vi "Abadines_server_sight.vi"() -> ()   [LabVIEW 2013]
uses:
  <vilib>/NXT/Block Support/NXT_InputPort.ctl
  <vilib>/NXT/Block Support/NXT_MessageMailbox.ctl
  <vilib>/NXT/Block Support/NXT_OutputPort.ctl
  <vilib>/NXT/Subs/MotorOutput.ctl
  <vilib>/NXT/Dual Mode Library/BT/BlueTooth_Write_Num.vi
  <vilib>/NXT/NXTIO Xnodes/NXTIONodeSubVIs/NXTStopMotors.vi
  <vilib>/NXT/Dual Mode Library/Display/drawNumber.vi
  <vilib>/NXT/Dual Mode Library/Display/drawNumber_float.vi
  <vilib>/NXT/NXTIO Xnodes/AddressXNode/NXTIOAddress.xnode
  <vilib>/NXT/NXTIO Xnodes/NXTIOXNode/NXTIO.xnode
  <vilib>/NXT/Subs/LVHSConnector.ctl
  <vilib>/NXT/LegoClasses/BrickReference/BrickReference.lvclass
panel:
  in  "threshold steer":dbl
  out "norm dist":dbl
  out "Blue Line":i16
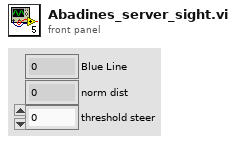
[diagram p1: front panel]
types:
  T1 = typedef "NXT_OutputPort.ctl" = u8
  T2 = typedef "NXT_InputPort.ctl" = u32
  T3 = typedef "LVHSConnector.ctl" = refnum<class "BrickReference.lvclass">
  T4 = typedef "NXT_MessageMailbox.ctl" = u8
  T5 = typedef "MotorOutput.ctl" = u8
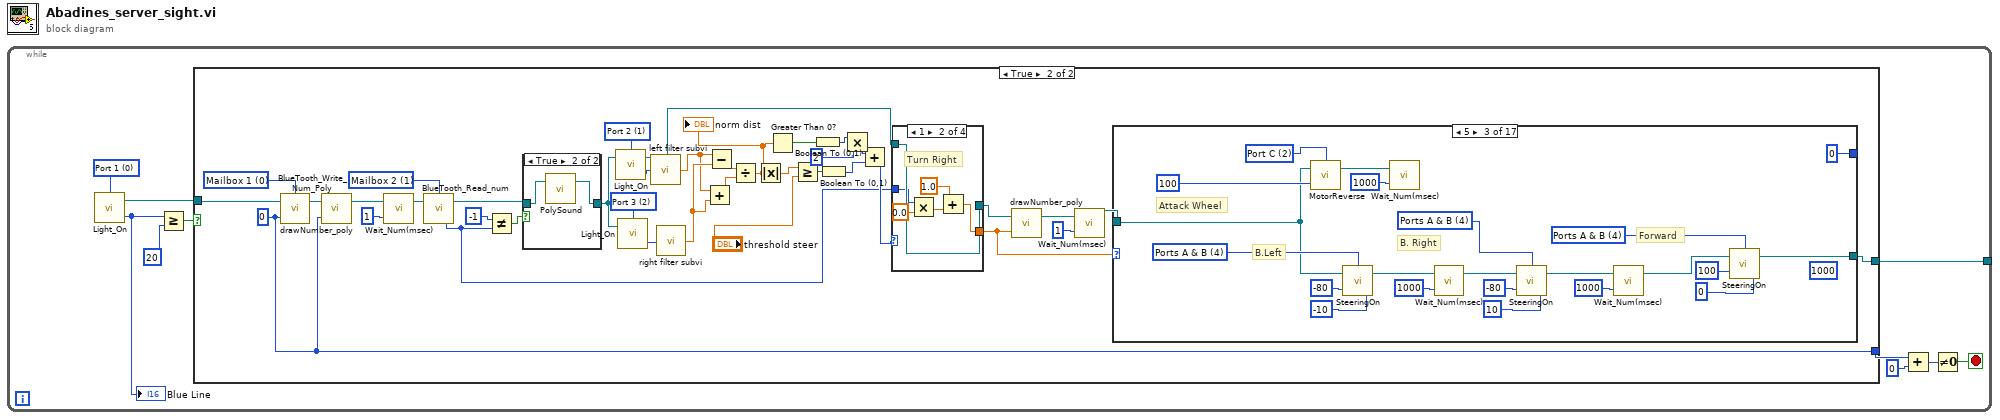
[diagram p0: block diagram]
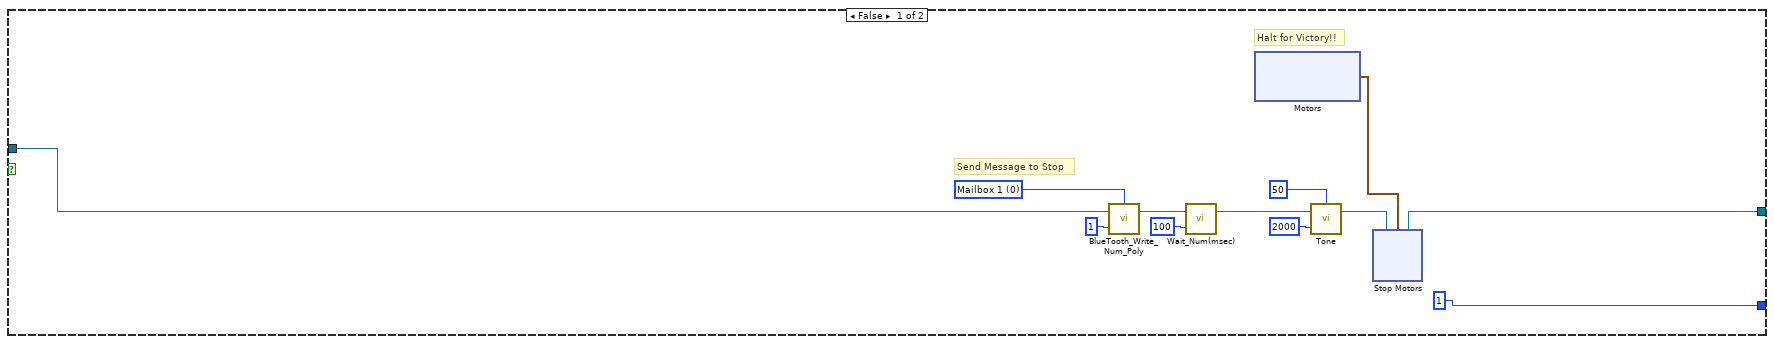
[diagram p2: hidden frame]
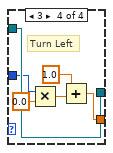
[diagram p5: hidden frame]
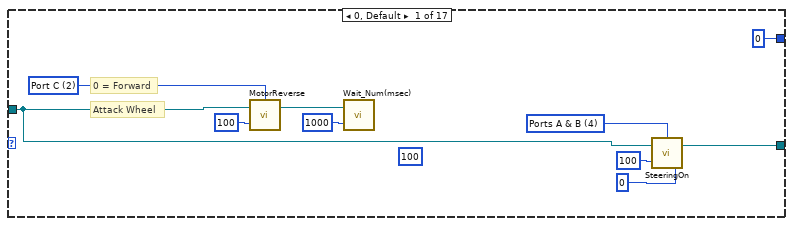
[diagram p7: hidden frame]
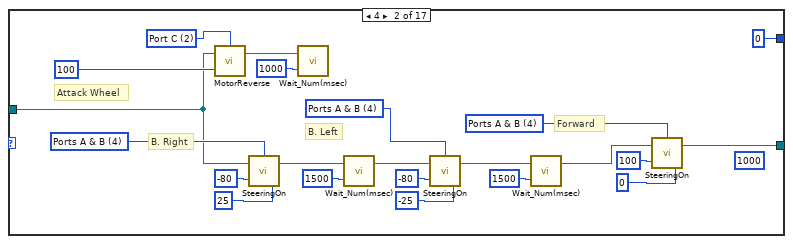
[diagram p8: hidden frame]
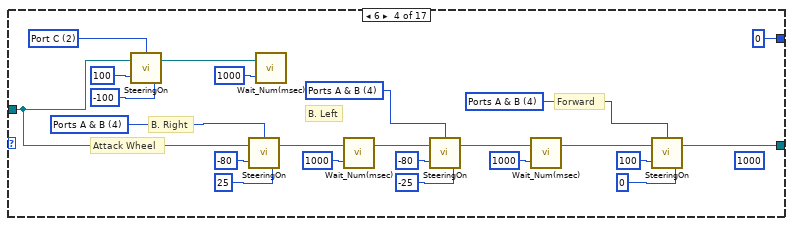
[diagram p9: hidden frame]
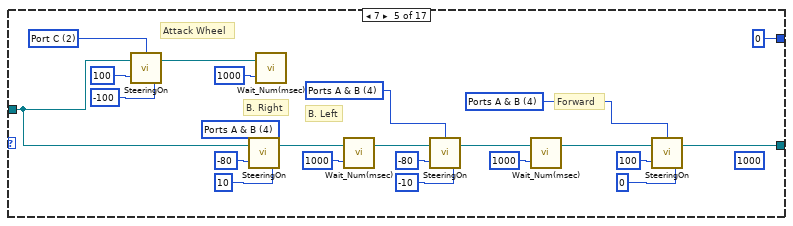
[diagram p10: hidden frame]
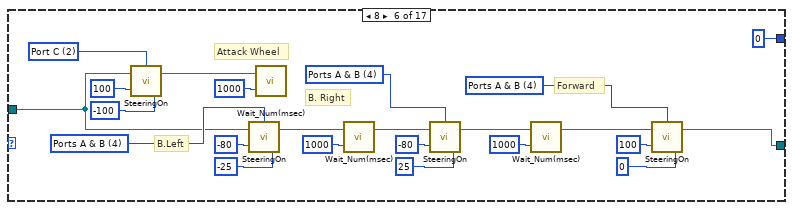
[diagram p11: hidden frame]
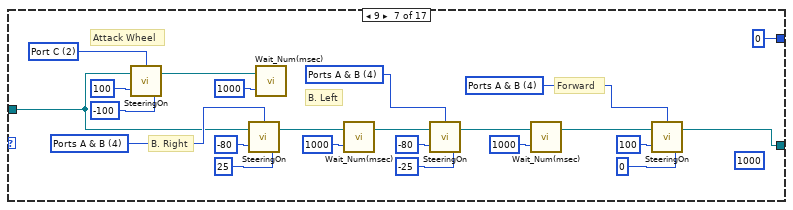
[diagram p12: hidden frame]
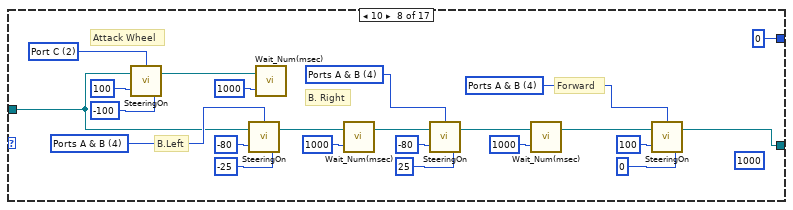
[diagram p13: hidden frame]
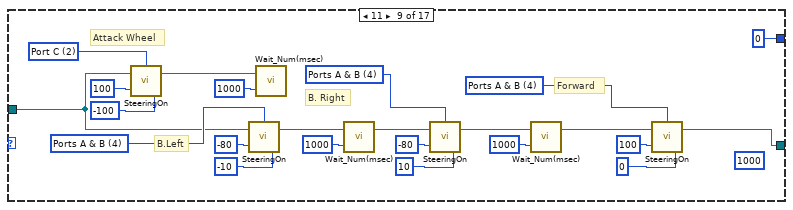
[diagram p14: hidden frame]
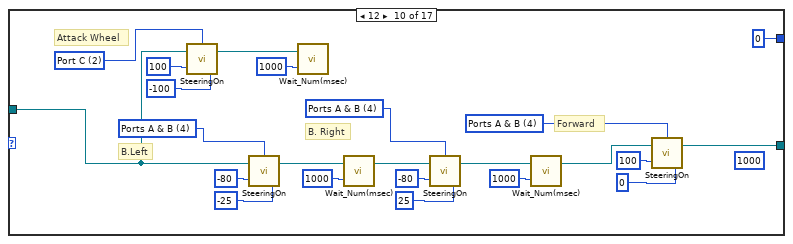
[diagram p15: hidden frame]
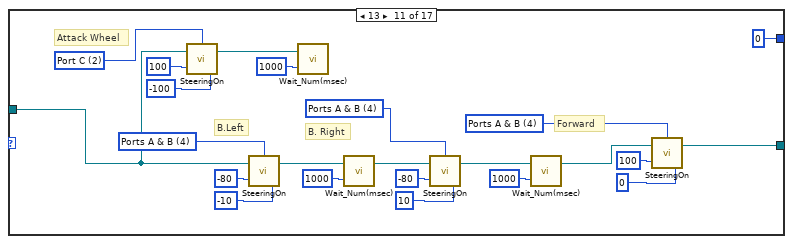
[diagram p16: hidden frame]
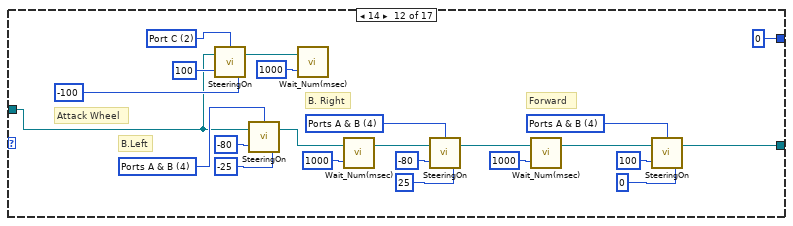
[diagram p17: hidden frame]
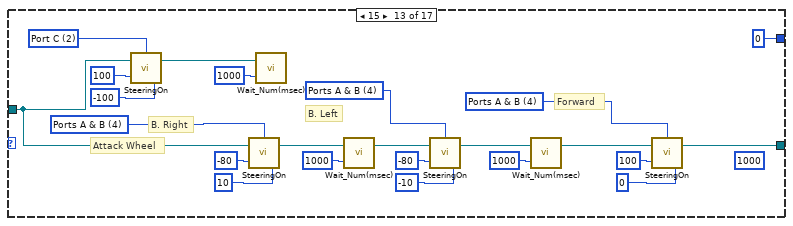
[diagram p18: hidden frame]
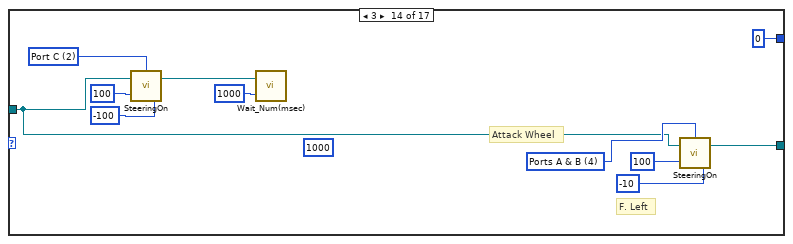
[diagram p19: hidden frame]
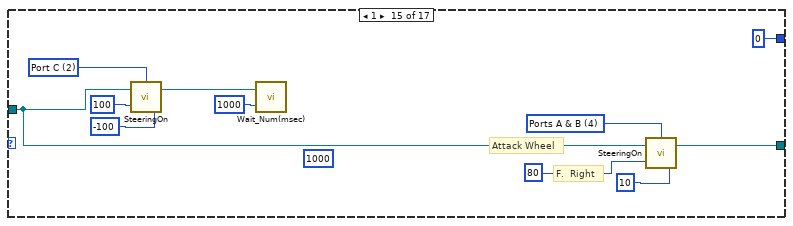
[diagram p20: hidden frame]
diagram:
  n1 = while {
    tunnel: [w6] -> _
    stop <- w2 stop-if-true
    w10 = T2 0 items=["Port 1", "Port 2", "Port 3", "Port 4"] ("Port (Port 3)")
    n2 = call <vilib>:"Light_On.vi"("Port (Port 3)"=w10) -> ("Scaled Value"=w9:i16, "NXT/EV3"=w1:T3)  [unwired: 2 in]
    "Blue Line" <- w9
    n3 = Greater Or Equal?(x=w9, y=i16 20) -> (x >= y?=w7:bool)
    n4 = case shown="True" w7 {
      tunnel: w1 -> [w20 w59]
      tunnel: [w14 w57] -> w6
      tunnel: [1 w56] -> w5
      frame False {
        w21 = T4 0 items=["Mailbox 1", "Mailbox 2", "Mailbox 3", "Mailbox 4", "Mailbox 5", "Mailbox 6", "Mailbox 7", "Mailbox 8", "Mailbox 9", "Mailbox 10"] ("Mailbox")
        # "Halt for Victory!!"
        # "Send Message to Stop"
        n5 = call-poly <vilib>:"BlueTooth_Write_Num_Poly.vi"("Message"=1, "NXT/EV3"=w20, "Mailbox"=w21) -> ("NXT/EV3"=w16:T3)  [unwired: 1 in]
        n6 = call <vilib>:"Wait_Num(msec).vi"("Time (100 msec)"=u32 100, "NXT/EV3"=w16) -> ("NXT/EV3"=w17:T3)  [unwired: 2 in]
        n7 = xnode "Motors"() -> ("Motor"=w13:cluster{"Port":T1, "Port":T1})
        n8 = call <vilib>:"Tone.vi"("Duration (500 ms)"=u16 2000, "NXT/EV3"=w17, "Tone (440 Hz)"=u16 50) -> ("NXT/EV3"=w15:T3)  [unwired: 1 in]
        n9 = xnode "Stop Motors"("Motors"=w13, "NXT/EV3"=w15) -> ("NXT/EV3"=w14:T3)
      }
      frame True {
        w50 = T2 2 items=["Port 1", "Port 2", "Port 3", "Port 4"] ("Port (Port 3)")
        w51 = T2 1 items=["Port 1", "Port 2", "Port 3", "Port 4"] ("Port (Port 3)")
        w66 = T4 1 items=["Mailbox 1", "Mailbox 2", "Mailbox 3", "Mailbox 4", "Mailbox 5", "Mailbox 6", "Mailbox 7", "Mailbox 8", "Mailbox 9", "Mailbox 10"] ("Mailbox")
        w56 = 0 ("Message")
        w60 = T4 0 items=["Mailbox 1", "Mailbox 2", "Mailbox 3", "Mailbox 4", "Mailbox 5", "Mailbox 6", "Mailbox 7", "Mailbox 8", "Mailbox 9", "Mailbox 10"] ("Mailbox")
        n10 = call-poly <vilib>:"BlueTooth_Write_Num_Poly.vi"("Message"=w56, "NXT/EV3"=w59, "Mailbox"=w60) -> ("NXT/EV3"=w53:T3)  [unwired: 1 in]
        n11 = call-poly <vilib>:"drawNumber_poly.vi"("number"=w56, "NXT/EV3"=w53) -> ("NXT/EV3"=w61:T3)  [unwired: 2 in]
        n12 = call <vilib>:"Wait_Num(msec).vi"("Time (100 msec)"=u32 1, "NXT/EV3"=w61) -> ("NXT/EV3"=w62:T3)  [unwired: 2 in]
        n13 = call <vilib>:"BlueTooth_Read_num.vi"("NXT/EV3"=w62, "Mailbox"=w66) -> ("Message"=w30:i32, "NXT/EV3"=w52:T3)  [unwired: 1 in]
        n14 = Not Equal?(x=-1, y=w30) -> (x != y?=w54:bool)
        n15 = case shown="True" w54 {
          tunnel: [w83 w85] -> w33
          tunnel: w52 -> [w83 w84]
          frame False {
          }
          frame True {
            n16 = call-poly <vilib>:"PolySound.vi"("NXT/EV3"=w84) -> ("NXT/EV3"=w85:T3)  [unwired: 3 in]
          }
        }
        n17 = call <vilib>:"Light_On.vi"("NXT/EV3"=w33, "Port (Port 3)"=w51) -> ("Scaled Value"=w48:i16, "NXT/EV3"=w32:T3)  [unwired: 1 in]
        n18 = call <vilib>:"Light_On.vi"("NXT/EV3"=w33, "Port (Port 3)"=w50) -> ("Scaled Value"=w49:i16)  [unwired: 1 in, 1 out]
        n19 = call "left filter subvi.vi"("raw value in"=w48) -> ("filtered signal"=w46:dbl)  [unwired: 14 in]
        n20 = call "right filter subvi.vi"("raw value in"=w49) -> ("filtered signal"=w47:dbl)  [unwired: 14 in]
        n21 = Add(x=w46, y=w47) -> (x+y=w44:dbl)
        n22 = Subtract(x=w46, y=w47) -> (x-y=w45:dbl)
        n23 = Divide(x=w45, y=w44) -> (x/y=w41:dbl)
        "norm dist" <- w41
        n24 = Absolute Value(x=w41) -> (abs(x)=w43:dbl)
        n25 = Greater Than 0?(x=w41) -> (x > 0?=w39:bool)
        n26 = Greater Or Equal?(x=w43, y="threshold steer") -> (x >= y?=w40:bool)
        n27 = Boolean To (0,1)(Boolean=w39) -> (0, 1=w38:i16)
        n28 = Boolean To (0,1)(Boolean=w40) -> (0, 1=w36:i16)
        n29 = Multiply(x=w38, y=i16 2) -> (x*y=w35:i16)
        n30 = Add(x=w35, y=w36) -> (x+y=w34:i16)
        n31 = case shown="1" w34 {
          tunnel: w32 -> [w68 w72 w76 w82]
          tunnel: [w68 w72 w76 w82] -> w31
          tunnel: w30 -> [w67 w71 w75 w78]
          tunnel: [w67 w70 w75 w77] -> w29
          frame 0, Default {
          }
          frame 1 {
            # "Turn Right"
            n32 = Multiply(x=w71, y=0.0) -> (x*y=w69:dbl)
            n33 = Add(x=1.0, y=w69) -> (x+y=w70:dbl)
          }
          frame 2 {
          }
          frame 3 {
            # "Turn Left"
            n34 = Multiply(x=w78, y=0.0) -> (x*y=w80:dbl)
            n35 = Add(x=1.0, y=w80) -> (x+y=w77:dbl)
          }
        }
        n36 = call-poly <vilib>:"drawNumber_poly.vi"("number"=w29, "NXT/EV3"=w31) -> ("NXT/EV3"=w65:T3)  [unwired: 2 in]
        n37 = call <vilib>:"Wait_Num(msec).vi"("Time (100 msec)"=u32 1, "NXT/EV3"=w65) -> ("NXT/EV3"=w58:T3)  [unwired: 2 in]
        n38 = case shown="5" w29 {
          tunnel: [w93 w111 w124 w147 w170 w202 w216 w239 w262 w286 w308 w331 w355 w378 w389 w398 w415] -> w57
          tunnel: w58 -> [w86 w96 w118 w140 w163 w186 w209 w232 w255 w279 w302 w324 w347 w370 w381 w394 w408]
          tunnel: [0 ("Steering (100)") 0 ("Steering (100)") 0 ("Steering (100)") 0 ("Steering (100)") 0 ("Steering (100)") 0 ("Steering (100)") 0 ("Steering (100)") 0 ("Steering (100)") 0 ("Steering (100)") 0 ("Steering (100)") 0 ("Steering (100)") 0 ("Steering (100)") 0 ("Steering (100)") 0 ("Steering (100)") 0 ("Steering (100)") 1 ("Steering (100)") 0 ("Steering (100)")] -> _
          frame 0, Default {
            (unwired) u16 100 ("Duration (500 ms)")
            w91 = T5 2 items=["Port A"=0, "Port B"=1, "Port C"=2, "Ports A & B"=4, "Ports A & C"=5, "Ports B & C"=6, "All Ports"=3] ("Output Ports (A & B)")
            w92 = T5 4 items=["Port A"=0, "Port B"=1, "Port C"=2, "Ports A & B"=4, "Ports A & C"=5, "Ports B & C"=6, "All Ports"=3] ("Output Ports (A & B) 5")
            # "Attack Wheel"
            # "0 = Forward"
            n39 = call <vilib>:"MotorReverse.vi"("Power (75)"=100, "NXT/EV3"=w86, "Output Port (All Ports)"=w91) -> ("NXT/EV3"=w89:T3)  [unwired: 1 in]
            n40 = call <vilib>:"Wait_Num(msec).vi"("Time (100 msec)"=u32 1000, "NXT/EV3"=w89) -> ()  [unwired: 2 in, 1 out]
            n41 = call <vilib>:"SteeringOn.vi"("Power (75)"=100, "Steering (100)"=0, "NXT/EV3"=w86, "Output Ports (A & B)"=w92) -> ("NXT/EV3"=w93:T3)
          }
          frame 4 {
            (unwired) u16 1000 ("Duration (500 ms)")
            w101 = T5 2 items=["Port A"=0, "Port B"=1, "Port C"=2, "Ports A & B"=4, "Ports A & C"=5, "Ports B & C"=6, "All Ports"=3] ("Output Ports (A & B)")
            w108 = T5 4 items=["Port A"=0, "Port B"=1, "Port C"=2, "Ports A & B"=4, "Ports A & C"=5, "Ports B & C"=6, "All Ports"=3] ("Output Ports (A & B) 15")
            w109 = T5 4 items=["Port A"=0, "Port B"=1, "Port C"=2, "Ports A & B"=4, "Ports A & C"=5, "Ports B & C"=6, "All Ports"=3] ("Output Port (All Ports) 6")
            w110 = T5 4 items=["Port A"=0, "Port B"=1, "Port C"=2, "Ports A & B"=4, "Ports A & C"=5, "Ports B & C"=6, "All Ports"=3] ("Output Ports (A & B) 16")
            # "Attack Wheel"
            # "Forward"
            # "B. Left"
            # "B. Right"
            n42 = call <vilib>:"MotorReverse.vi"("Power (75)"=100, "NXT/EV3"=w96, "Output Port (All Ports)"=w101) -> ("NXT/EV3"=w99:T3)  [unwired: 1 in]
            n43 = call <vilib>:"SteeringOn.vi"("Power (75)"=-80, "Steering (100)"=25, "NXT/EV3"=w96, "Output Ports (A & B)"=w110) -> ("NXT/EV3"=w107:T3)
            n44 = call <vilib>:"Wait_Num(msec).vi"("Time (100 msec)"=u32 1000, "NXT/EV3"=w99) -> ()  [unwired: 2 in, 1 out]
            n45 = call <vilib>:"Wait_Num(msec).vi"("Time (100 msec)"=u32 1500, "NXT/EV3"=w107) -> ("NXT/EV3"=w106:T3)  [unwired: 2 in]
            n46 = call <vilib>:"SteeringOn.vi"("Power (75)"=-80, "Steering (100)"=-25, "NXT/EV3"=w106, "Output Ports (A & B)"=w109) -> ("NXT/EV3"=w105:T3)
            n47 = call <vilib>:"Wait_Num(msec).vi"("Time (100 msec)"=u32 1500, "NXT/EV3"=w105) -> ("NXT/EV3"=w104:T3)  [unwired: 2 in]
            n48 = call <vilib>:"SteeringOn.vi"("Power (75)"=100, "Steering (100)"=0, "NXT/EV3"=w104, "Output Ports (A & B)"=w108) -> ("NXT/EV3"=w111:T3)
          }
          frame 5 {
            (unwired) u16 1000 ("Duration (500 ms)")
            w123 = T5 2 items=["Port A"=0, "Port B"=1, "Port C"=2, "Ports A & B"=4, "Ports A & C"=5, "Ports B & C"=6, "All Ports"=3] ("Output Ports (A & B)")
            w131 = T5 4 items=["Port A"=0, "Port B"=1, "Port C"=2, "Ports A & B"=4, "Ports A & C"=5, "Ports B & C"=6, "All Ports"=3] ("Output Ports (A & B) 21")
            w132 = T5 4 items=["Port A"=0, "Port B"=1, "Port C"=2, "Ports A & B"=4, "Ports A & C"=5, "Ports B & C"=6, "All Ports"=3] ("Output Port (All Ports) 9")
            w133 = T5 4 items=["Port A"=0, "Port B"=1, "Port C"=2, "Ports A & B"=4, "Ports A & C"=5, "Ports B & C"=6, "All Ports"=3] ("Output Ports (A & B) 22")
            # "Attack Wheel"
            # "Forward"
            # "B. Right"
            # "B.Left"
            n49 = call <vilib>:"MotorReverse.vi"("Power (75)"=100, "NXT/EV3"=w118, "Output Port (All Ports)"=w123) -> ("NXT/EV3"=w121:T3)  [unwired: 1 in]
            n50 = call <vilib>:"SteeringOn.vi"("Power (75)"=-80, "Steering (100)"=-10, "NXT/EV3"=w118, "Output Ports (A & B)"=w133) -> ("NXT/EV3"=w129:T3)
            n51 = call <vilib>:"Wait_Num(msec).vi"("Time (100 msec)"=u32 1000, "NXT/EV3"=w121) -> ()  [unwired: 2 in, 1 out]
            n52 = call <vilib>:"Wait_Num(msec).vi"("Time (100 msec)"=u32 1000, "NXT/EV3"=w129) -> ("NXT/EV3"=w128:T3)  [unwired: 2 in]
            n53 = call <vilib>:"SteeringOn.vi"("Power (75)"=-80, "Steering (100)"=10, "NXT/EV3"=w128, "Output Ports (A & B)"=w132) -> ("NXT/EV3"=w126:T3)
            n54 = call <vilib>:"Wait_Num(msec).vi"("Time (100 msec)"=u32 1000, "NXT/EV3"=w126) -> ("NXT/EV3"=w125:T3)  [unwired: 2 in]
            n55 = call <vilib>:"SteeringOn.vi"("Power (75)"=100, "Steering (100)"=0, "NXT/EV3"=w125, "Output Ports (A & B)"=w131) -> ("NXT/EV3"=w124:T3)
          }
          frame 6 {
            (unwired) u16 1000 ("Duration (500 ms)")
            w146 = T5 2 items=["Port A"=0, "Port B"=1, "Port C"=2, "Ports A & B"=4, "Ports A & C"=5, "Ports B & C"=6, "All Ports"=3] ("Output Ports (A & B)")
            w156 = T5 4 items=["Port A"=0, "Port B"=1, "Port C"=2, "Ports A & B"=4, "Ports A & C"=5, "Ports B & C"=6, "All Ports"=3] ("Output Ports (A & B) 15")
            w155 = T5 4 items=["Port A"=0, "Port B"=1, "Port C"=2, "Ports A & B"=4, "Ports A & C"=5, "Ports B & C"=6, "All Ports"=3] ("Output Port (All Ports) 6")
            w154 = T5 4 items=["Port A"=0, "Port B"=1, "Port C"=2, "Ports A & B"=4, "Ports A & C"=5, "Ports B & C"=6, "All Ports"=3] ("Output Ports (A & B) 16")
            # "Attack Wheel"
            # "Forward"
            # "B. Left"
            # "B. Right"
            n56 = call <vilib>:"SteeringOn.vi"("Power (75)"=100, "Steering (100)"=-100, "NXT/EV3"=w140, "Output Ports (A & B)"=w146) -> ("NXT/EV3"=w143:T3)
            n57 = call <vilib>:"SteeringOn.vi"("Power (75)"=-80, "Steering (100)"=25, "NXT/EV3"=w140, "Output Ports (A & B)"=w154) -> ("NXT/EV3"=w157:T3)
            n58 = call <vilib>:"Wait_Num(msec).vi"("Time (100 msec)"=u32 1000, "NXT/EV3"=w143) -> ()  [unwired: 2 in, 1 out]
            n59 = call <vilib>:"Wait_Num(msec).vi"("Time (100 msec)"=u32 1000, "NXT/EV3"=w157) -> ("NXT/EV3"=w158:T3)  [unwired: 2 in]
            n60 = call <vilib>:"SteeringOn.vi"("Power (75)"=-80, "Steering (100)"=-25, "NXT/EV3"=w158, "Output Ports (A & B)"=w155) -> ("NXT/EV3"=w159:T3)
            n61 = call <vilib>:"Wait_Num(msec).vi"("Time (100 msec)"=u32 1000, "NXT/EV3"=w159) -> ("NXT/EV3"=w160:T3)  [unwired: 2 in]
            n62 = call <vilib>:"SteeringOn.vi"("Power (75)"=100, "Steering (100)"=0, "NXT/EV3"=w160, "Output Ports (A & B)"=w156) -> ("NXT/EV3"=w147:T3)
          }
          frame 7 {
            (unwired) u16 1000 ("Duration (500 ms)")
            w169 = T5 2 items=["Port A"=0, "Port B"=1, "Port C"=2, "Ports A & B"=4, "Ports A & C"=5, "Ports B & C"=6, "All Ports"=3] ("Output Ports (A & B)")
            w179 = T5 4 items=["Port A"=0, "Port B"=1, "Port C"=2, "Ports A & B"=4, "Ports A & C"=5, "Ports B & C"=6, "All Ports"=3] ("Output Ports (A & B) 15")
            w178 = T5 4 items=["Port A"=0, "Port B"=1, "Port C"=2, "Ports A & B"=4, "Ports A & C"=5, "Ports B & C"=6, "All Ports"=3] ("Output Port (All Ports) 6")
            w177 = T5 4 items=["Port A"=0, "Port B"=1, "Port C"=2, "Ports A & B"=4, "Ports A & C"=5, "Ports B & C"=6, "All Ports"=3] ("Output Ports (A & B) 16")
            # "Attack Wheel"
            # "Forward"
            # "B. Left"
            # "B. Right"
            n63 = call <vilib>:"SteeringOn.vi"("Power (75)"=100, "Steering (100)"=-100, "NXT/EV3"=w163, "Output Ports (A & B)"=w169) -> ("NXT/EV3"=w166:T3)
            n64 = call <vilib>:"SteeringOn.vi"("Power (75)"=-80, "Steering (100)"=10, "NXT/EV3"=w163, "Output Ports (A & B)"=w177) -> ("NXT/EV3"=w180:T3)
            n65 = call <vilib>:"Wait_Num(msec).vi"("Time (100 msec)"=u32 1000, "NXT/EV3"=w166) -> ()  [unwired: 2 in, 1 out]
            n66 = call <vilib>:"Wait_Num(msec).vi"("Time (100 msec)"=u32 1000, "NXT/EV3"=w180) -> ("NXT/EV3"=w181:T3)  [unwired: 2 in]
            n67 = call <vilib>:"SteeringOn.vi"("Power (75)"=-80, "Steering (100)"=-10, "NXT/EV3"=w181, "Output Ports (A & B)"=w178) -> ("NXT/EV3"=w182:T3)
            n68 = call <vilib>:"Wait_Num(msec).vi"("Time (100 msec)"=u32 1000, "NXT/EV3"=w182) -> ("NXT/EV3"=w183:T3)  [unwired: 2 in]
            n69 = call <vilib>:"SteeringOn.vi"("Power (75)"=100, "Steering (100)"=0, "NXT/EV3"=w183, "Output Ports (A & B)"=w179) -> ("NXT/EV3"=w170:T3)
          }
          frame 8 {
            w192 = T5 2 items=["Port A"=0, "Port B"=1, "Port C"=2, "Ports A & B"=4, "Ports A & C"=5, "Ports B & C"=6, "All Ports"=3] ("Output Ports (A & B)")
            w199 = T5 4 items=["Port A"=0, "Port B"=1, "Port C"=2, "Ports A & B"=4, "Ports A & C"=5, "Ports B & C"=6, "All Ports"=3] ("Output Ports (A & B) 21")
            w200 = T5 4 items=["Port A"=0, "Port B"=1, "Port C"=2, "Ports A & B"=4, "Ports A & C"=5, "Ports B & C"=6, "All Ports"=3] ("Output Port (All Ports) 9")
            w201 = T5 4 items=["Port A"=0, "Port B"=1, "Port C"=2, "Ports A & B"=4, "Ports A & C"=5, "Ports B & C"=6, "All Ports"=3] ("Output Ports (A & B) 22")
            # "Attack Wheel"
            # "Forward"
            # "B. Right"
            # "B.Left"
            n70 = call <vilib>:"SteeringOn.vi"("Power (75)"=100, "Steering (100)"=-100, "NXT/EV3"=w186, "Output Ports (A & B)"=w192) -> ("NXT/EV3"=w189:T3)
            n71 = call <vilib>:"SteeringOn.vi"("Power (75)"=-80, "Steering (100)"=-25, "NXT/EV3"=w186, "Output Ports (A & B)"=w201) -> ("NXT/EV3"=w197:T3)
            n72 = call <vilib>:"Wait_Num(msec).vi"("Time (100 msec)"=u32 1000, "NXT/EV3"=w189) -> ()  [unwired: 2 in, 1 out]
            n73 = call <vilib>:"Wait_Num(msec).vi"("Time (100 msec)"=u32 1000, "NXT/EV3"=w197) -> ("NXT/EV3"=w196:T3)  [unwired: 2 in]
            n74 = call <vilib>:"SteeringOn.vi"("Power (75)"=-80, "Steering (100)"=25, "NXT/EV3"=w196, "Output Ports (A & B)"=w200) -> ("NXT/EV3"=w194:T3)
            n75 = call <vilib>:"Wait_Num(msec).vi"("Time (100 msec)"=u32 1000, "NXT/EV3"=w194) -> ("NXT/EV3"=w193:T3)  [unwired: 2 in]
            n76 = call <vilib>:"SteeringOn.vi"("Power (75)"=100, "Steering (100)"=0, "NXT/EV3"=w193, "Output Ports (A & B)"=w199) -> ("NXT/EV3"=w202:T3)
          }
          frame 9 {
            (unwired) u16 1000 ("Duration (500 ms)")
            w215 = T5 2 items=["Port A"=0, "Port B"=1, "Port C"=2, "Ports A & B"=4, "Ports A & C"=5, "Ports B & C"=6, "All Ports"=3] ("Output Ports (A & B)")
            w223 = T5 4 items=["Port A"=0, "Port B"=1, "Port C"=2, "Ports A & B"=4, "Ports A & C"=5, "Ports B & C"=6, "All Ports"=3] ("Output Ports (A & B) 15")
            w224 = T5 4 items=["Port A"=0, "Port B"=1, "Port C"=2, "Ports A & B"=4, "Ports A & C"=5, "Ports B & C"=6, "All Ports"=3] ("Output Port (All Ports) 6")
            w225 = T5 4 items=["Port A"=0, "Port B"=1, "Port C"=2, "Ports A & B"=4, "Ports A & C"=5, "Ports B & C"=6, "All Ports"=3] ("Output Ports (A & B) 16")
            # "Attack Wheel"
            # "Forward"
            # "B. Left"
            # "B. Right"
            n77 = call <vilib>:"SteeringOn.vi"("Power (75)"=100, "Steering (100)"=-100, "NXT/EV3"=w209, "Output Ports (A & B)"=w215) -> ("NXT/EV3"=w212:T3)
            n78 = call <vilib>:"SteeringOn.vi"("Power (75)"=-80, "Steering (100)"=25, "NXT/EV3"=w209, "Output Ports (A & B)"=w225) -> ("NXT/EV3"=w222:T3)
            n79 = call <vilib>:"Wait_Num(msec).vi"("Time (100 msec)"=u32 1000, "NXT/EV3"=w212) -> ()  [unwired: 2 in, 1 out]
            n80 = call <vilib>:"Wait_Num(msec).vi"("Time (100 msec)"=u32 1000, "NXT/EV3"=w222) -> ("NXT/EV3"=w221:T3)  [unwired: 2 in]
            n81 = call <vilib>:"SteeringOn.vi"("Power (75)"=-80, "Steering (100)"=-25, "NXT/EV3"=w221, "Output Ports (A & B)"=w224) -> ("NXT/EV3"=w220:T3)
            n82 = call <vilib>:"Wait_Num(msec).vi"("Time (100 msec)"=u32 1000, "NXT/EV3"=w220) -> ("NXT/EV3"=w219:T3)  [unwired: 2 in]
            n83 = call <vilib>:"SteeringOn.vi"("Power (75)"=100, "Steering (100)"=0, "NXT/EV3"=w219, "Output Ports (A & B)"=w223) -> ("NXT/EV3"=w216:T3)
          }
          frame 10 {
            (unwired) u16 1000 ("Duration (500 ms)")
            w238 = T5 2 items=["Port A"=0, "Port B"=1, "Port C"=2, "Ports A & B"=4, "Ports A & C"=5, "Ports B & C"=6, "All Ports"=3] ("Output Ports (A & B)")
            w248 = T5 4 items=["Port A"=0, "Port B"=1, "Port C"=2, "Ports A & B"=4, "Ports A & C"=5, "Ports B & C"=6, "All Ports"=3] ("Output Ports (A & B) 21")
            w247 = T5 4 items=["Port A"=0, "Port B"=1, "Port C"=2, "Ports A & B"=4, "Ports A & C"=5, "Ports B & C"=6, "All Ports"=3] ("Output Port (All Ports) 9")
            w246 = T5 4 items=["Port A"=0, "Port B"=1, "Port C"=2, "Ports A & B"=4, "Ports A & C"=5, "Ports B & C"=6, "All Ports"=3] ("Output Ports (A & B) 22")
            # "Attack Wheel"
            # "Forward"
            # "B. Right"
            # "B.Left"
            n84 = call <vilib>:"SteeringOn.vi"("Power (75)"=100, "Steering (100)"=-100, "NXT/EV3"=w232, "Output Ports (A & B)"=w238) -> ("NXT/EV3"=w235:T3)
            n85 = call <vilib>:"SteeringOn.vi"("Power (75)"=-80, "Steering (100)"=-25, "NXT/EV3"=w232, "Output Ports (A & B)"=w246) -> ("NXT/EV3"=w250:T3)
            n86 = call <vilib>:"Wait_Num(msec).vi"("Time (100 msec)"=u32 1000, "NXT/EV3"=w235) -> ()  [unwired: 2 in, 1 out]
            n87 = call <vilib>:"Wait_Num(msec).vi"("Time (100 msec)"=u32 1000, "NXT/EV3"=w250) -> ("NXT/EV3"=w251:T3)  [unwired: 2 in]
            n88 = call <vilib>:"SteeringOn.vi"("Power (75)"=-80, "Steering (100)"=25, "NXT/EV3"=w251, "Output Ports (A & B)"=w247) -> ("NXT/EV3"=w253:T3)
            n89 = call <vilib>:"Wait_Num(msec).vi"("Time (100 msec)"=u32 1000, "NXT/EV3"=w253) -> ("NXT/EV3"=w254:T3)  [unwired: 2 in]
            n90 = call <vilib>:"SteeringOn.vi"("Power (75)"=100, "Steering (100)"=0, "NXT/EV3"=w254, "Output Ports (A & B)"=w248) -> ("NXT/EV3"=w239:T3)
          }
          frame 11 {
            (unwired) u16 1000 ("Duration (500 ms)")
            w261 = T5 2 items=["Port A"=0, "Port B"=1, "Port C"=2, "Ports A & B"=4, "Ports A & C"=5, "Ports B & C"=6, "All Ports"=3] ("Output Ports (A & B)")
            w271 = T5 4 items=["Port A"=0, "Port B"=1, "Port C"=2, "Ports A & B"=4, "Ports A & C"=5, "Ports B & C"=6, "All Ports"=3] ("Output Ports (A & B) 21")
            w270 = T5 4 items=["Port A"=0, "Port B"=1, "Port C"=2, "Ports A & B"=4, "Ports A & C"=5, "Ports B & C"=6, "All Ports"=3] ("Output Port (All Ports) 9")
            w269 = T5 4 items=["Port A"=0, "Port B"=1, "Port C"=2, "Ports A & B"=4, "Ports A & C"=5, "Ports B & C"=6, "All Ports"=3] ("Output Ports (A & B) 22")
            # "Attack Wheel"
            # "Forward"
            # "B. Right"
            # "B.Left"
            n91 = call <vilib>:"SteeringOn.vi"("Power (75)"=100, "Steering (100)"=-100, "NXT/EV3"=w255, "Output Ports (A & B)"=w261) -> ("NXT/EV3"=w258:T3)
            n92 = call <vilib>:"SteeringOn.vi"("Power (75)"=-80, "Steering (100)"=-10, "NXT/EV3"=w255, "Output Ports (A & B)"=w269) -> ("NXT/EV3"=w273:T3)
            n93 = call <vilib>:"Wait_Num(msec).vi"("Time (100 msec)"=u32 1000, "NXT/EV3"=w258) -> ()  [unwired: 2 in, 1 out]
            n94 = call <vilib>:"Wait_Num(msec).vi"("Time (100 msec)"=u32 1000, "NXT/EV3"=w273) -> ("NXT/EV3"=w274:T3)  [unwired: 2 in]
            n95 = call <vilib>:"SteeringOn.vi"("Power (75)"=-80, "Steering (100)"=10, "NXT/EV3"=w274, "Output Ports (A & B)"=w270) -> ("NXT/EV3"=w276:T3)
            n96 = call <vilib>:"Wait_Num(msec).vi"("Time (100 msec)"=u32 1000, "NXT/EV3"=w276) -> ("NXT/EV3"=w277:T3)  [unwired: 2 in]
            n97 = call <vilib>:"SteeringOn.vi"("Power (75)"=100, "Steering (100)"=0, "NXT/EV3"=w277, "Output Ports (A & B)"=w271) -> ("NXT/EV3"=w262:T3)
          }
          frame 12 {
            (unwired) u16 1000 ("Duration (500 ms)")
            w285 = T5 2 items=["Port A"=0, "Port B"=1, "Port C"=2, "Ports A & B"=4, "Ports A & C"=5, "Ports B & C"=6, "All Ports"=3] ("Output Ports (A & B)")
            w294 = T5 4 items=["Port A"=0, "Port B"=1, "Port C"=2, "Ports A & B"=4, "Ports A & C"=5, "Ports B & C"=6, "All Ports"=3] ("Output Ports (A & B) 21")
            w293 = T5 4 items=["Port A"=0, "Port B"=1, "Port C"=2, "Ports A & B"=4, "Ports A & C"=5, "Ports B & C"=6, "All Ports"=3] ("Output Port (All Ports) 9")
            w278 = T5 4 items=["Port A"=0, "Port B"=1, "Port C"=2, "Ports A & B"=4, "Ports A & C"=5, "Ports B & C"=6, "All Ports"=3] ("Output Ports (A & B) 22")
            # "Attack Wheel"
            # "Forward"
            # "B. Right"
            # "B.Left"
            n98 = call <vilib>:"SteeringOn.vi"("Power (75)"=100, "Steering (100)"=-100, "NXT/EV3"=w279, "Output Ports (A & B)"=w285) -> ("NXT/EV3"=w282:T3)
            n99 = call <vilib>:"SteeringOn.vi"("Power (75)"=-80, "Steering (100)"=-25, "NXT/EV3"=w279, "Output Ports (A & B)"=w278) -> ("NXT/EV3"=w296:T3)
            n100 = call <vilib>:"Wait_Num(msec).vi"("Time (100 msec)"=u32 1000, "NXT/EV3"=w282) -> ()  [unwired: 2 in, 1 out]
            n101 = call <vilib>:"Wait_Num(msec).vi"("Time (100 msec)"=u32 1000, "NXT/EV3"=w296) -> ("NXT/EV3"=w297:T3)  [unwired: 2 in]
            n102 = call <vilib>:"SteeringOn.vi"("Power (75)"=-80, "Steering (100)"=25, "NXT/EV3"=w297, "Output Ports (A & B)"=w293) -> ("NXT/EV3"=w299:T3)
            n103 = call <vilib>:"Wait_Num(msec).vi"("Time (100 msec)"=u32 1000, "NXT/EV3"=w299) -> ("NXT/EV3"=w300:T3)  [unwired: 2 in]
            n104 = call <vilib>:"SteeringOn.vi"("Power (75)"=100, "Steering (100)"=0, "NXT/EV3"=w300, "Output Ports (A & B)"=w294) -> ("NXT/EV3"=w286:T3)
          }
          frame 13 {
            w307 = T5 2 items=["Port A"=0, "Port B"=1, "Port C"=2, "Ports A & B"=4, "Ports A & C"=5, "Ports B & C"=6, "All Ports"=3] ("Output Ports (A & B)")
            w315 = T5 4 items=["Port A"=0, "Port B"=1, "Port C"=2, "Ports A & B"=4, "Ports A & C"=5, "Ports B & C"=6, "All Ports"=3] ("Output Ports (A & B) 21")
            w316 = T5 4 items=["Port A"=0, "Port B"=1, "Port C"=2, "Ports A & B"=4, "Ports A & C"=5, "Ports B & C"=6, "All Ports"=3] ("Output Port (All Ports) 9")
            w317 = T5 4 items=["Port A"=0, "Port B"=1, "Port C"=2, "Ports A & B"=4, "Ports A & C"=5, "Ports B & C"=6, "All Ports"=3] ("Output Ports (A & B) 22")
            # "Attack Wheel"
            # "Forward"
            # "B. Right"
            # "B.Left"
            n105 = call <vilib>:"SteeringOn.vi"("Power (75)"=100, "Steering (100)"=-100, "NXT/EV3"=w302, "Output Ports (A & B)"=w307) -> ("NXT/EV3"=w304:T3)
            n106 = call <vilib>:"SteeringOn.vi"("Power (75)"=-80, "Steering (100)"=-10, "NXT/EV3"=w302, "Output Ports (A & B)"=w317) -> ("NXT/EV3"=w313:T3)
            n107 = call <vilib>:"Wait_Num(msec).vi"("Time (100 msec)"=u32 1000, "NXT/EV3"=w304) -> ()  [unwired: 2 in, 1 out]
            n108 = call <vilib>:"Wait_Num(msec).vi"("Time (100 msec)"=u32 1000, "NXT/EV3"=w313) -> ("NXT/EV3"=w312:T3)  [unwired: 2 in]
            n109 = call <vilib>:"SteeringOn.vi"("Power (75)"=-80, "Steering (100)"=10, "NXT/EV3"=w312, "Output Ports (A & B)"=w316) -> ("NXT/EV3"=w310:T3)
            n110 = call <vilib>:"Wait_Num(msec).vi"("Time (100 msec)"=u32 1000, "NXT/EV3"=w310) -> ("NXT/EV3"=w309:T3)  [unwired: 2 in]
            n111 = call <vilib>:"SteeringOn.vi"("Power (75)"=100, "Steering (100)"=0, "NXT/EV3"=w309, "Output Ports (A & B)"=w315) -> ("NXT/EV3"=w308:T3)
          }
          frame 14 {
            w330 = T5 2 items=["Port A"=0, "Port B"=1, "Port C"=2, "Ports A & B"=4, "Ports A & C"=5, "Ports B & C"=6, "All Ports"=3] ("Output Ports (A & B)")
            w340 = T5 4 items=["Port A"=0, "Port B"=1, "Port C"=2, "Ports A & B"=4, "Ports A & C"=5, "Ports B & C"=6, "All Ports"=3] ("Output Ports (A & B) 21")
            w339 = T5 4 items=["Port A"=0, "Port B"=1, "Port C"=2, "Ports A & B"=4, "Ports A & C"=5, "Ports B & C"=6, "All Ports"=3] ("Output Port (All Ports) 9")
            w338 = T5 4 items=["Port A"=0, "Port B"=1, "Port C"=2, "Ports A & B"=4, "Ports A & C"=5, "Ports B & C"=6, "All Ports"=3] ("Output Ports (A & B) 22")
            # "Attack Wheel"
            # "Forward"
            # "B. Right"
            # "B.Left"
            n112 = call <vilib>:"SteeringOn.vi"("Power (75)"=100, "Steering (100)"=-100, "NXT/EV3"=w324, "Output Ports (A & B)"=w330) -> ("NXT/EV3"=w327:T3)
            n113 = call <vilib>:"SteeringOn.vi"("Power (75)"=-80, "Steering (100)"=-25, "NXT/EV3"=w324, "Output Ports (A & B)"=w338) -> ("NXT/EV3"=w342:T3)
            n114 = call <vilib>:"Wait_Num(msec).vi"("Time (100 msec)"=u32 1000, "NXT/EV3"=w327) -> ()  [unwired: 2 in, 1 out]
            n115 = call <vilib>:"Wait_Num(msec).vi"("Time (100 msec)"=u32 1000, "NXT/EV3"=w342) -> ("NXT/EV3"=w343:T3)  [unwired: 2 in]
            n116 = call <vilib>:"SteeringOn.vi"("Power (75)"=-80, "Steering (100)"=25, "NXT/EV3"=w343, "Output Ports (A & B)"=w339) -> ("NXT/EV3"=w345:T3)
            n117 = call <vilib>:"Wait_Num(msec).vi"("Time (100 msec)"=u32 1000, "NXT/EV3"=w345) -> ("NXT/EV3"=w346:T3)  [unwired: 2 in]
            n118 = call <vilib>:"SteeringOn.vi"("Power (75)"=100, "Steering (100)"=0, "NXT/EV3"=w346, "Output Ports (A & B)"=w340) -> ("NXT/EV3"=w331:T3)
          }
          frame 15 {
            (unwired) u16 1000 ("Duration (500 ms)")
            w353 = T5 2 items=["Port A"=0, "Port B"=1, "Port C"=2, "Ports A & B"=4, "Ports A & C"=5, "Ports B & C"=6, "All Ports"=3] ("Output Ports (A & B)")
            w362 = T5 4 items=["Port A"=0, "Port B"=1, "Port C"=2, "Ports A & B"=4, "Ports A & C"=5, "Ports B & C"=6, "All Ports"=3] ("Output Ports (A & B) 15")
            w363 = T5 4 items=["Port A"=0, "Port B"=1, "Port C"=2, "Ports A & B"=4, "Ports A & C"=5, "Ports B & C"=6, "All Ports"=3] ("Output Port (All Ports) 6")
            w354 = T5 4 items=["Port A"=0, "Port B"=1, "Port C"=2, "Ports A & B"=4, "Ports A & C"=5, "Ports B & C"=6, "All Ports"=3] ("Output Ports (A & B) 16")
            # "Attack Wheel"
            # "Forward"
            # "B. Left"
            # "B. Right"
            n119 = call <vilib>:"SteeringOn.vi"("Power (75)"=100, "Steering (100)"=-100, "NXT/EV3"=w347, "Output Ports (A & B)"=w353) -> ("NXT/EV3"=w350:T3)
            n120 = call <vilib>:"SteeringOn.vi"("Power (75)"=-80, "Steering (100)"=10, "NXT/EV3"=w347, "Output Ports (A & B)"=w354) -> ("NXT/EV3"=w361:T3)
            n121 = call <vilib>:"Wait_Num(msec).vi"("Time (100 msec)"=u32 1000, "NXT/EV3"=w350) -> ()  [unwired: 2 in, 1 out]
            n122 = call <vilib>:"Wait_Num(msec).vi"("Time (100 msec)"=u32 1000, "NXT/EV3"=w361) -> ("NXT/EV3"=w360:T3)  [unwired: 2 in]
            n123 = call <vilib>:"SteeringOn.vi"("Power (75)"=-80, "Steering (100)"=-10, "NXT/EV3"=w360, "Output Ports (A & B)"=w363) -> ("NXT/EV3"=w359:T3)
            n124 = call <vilib>:"Wait_Num(msec).vi"("Time (100 msec)"=u32 1000, "NXT/EV3"=w359) -> ("NXT/EV3"=w358:T3)  [unwired: 2 in]
            n125 = call <vilib>:"SteeringOn.vi"("Power (75)"=100, "Steering (100)"=0, "NXT/EV3"=w358, "Output Ports (A & B)"=w362) -> ("NXT/EV3"=w355:T3)
          }
          frame 3 {
            (unwired) u16 1000 ("Duration (500 ms)")
            w376 = T5 2 items=["Port A"=0, "Port B"=1, "Port C"=2, "Ports A & B"=4, "Ports A & C"=5, "Ports B & C"=6, "All Ports"=3] ("Output Ports (A & B)")
            w377 = T5 4 items=["Port A"=0, "Port B"=1, "Port C"=2, "Ports A & B"=4, "Ports A & C"=5, "Ports B & C"=6, "All Ports"=3] ("Output Port (All Ports) 3")
            # "Attack Wheel"
            # "F. Left"
            n126 = call <vilib>:"SteeringOn.vi"("Power (75)"=100, "Steering (100)"=-100, "NXT/EV3"=w370, "Output Ports (A & B)"=w376) -> ("NXT/EV3"=w373:T3)
            n127 = call <vilib>:"Wait_Num(msec).vi"("Time (100 msec)"=u32 1000, "NXT/EV3"=w373) -> ()  [unwired: 2 in, 1 out]
            n128 = call <vilib>:"SteeringOn.vi"("Power (75)"=100, "Steering (100)"=-10, "NXT/EV3"=w370, "Output Ports (A & B)"=w377) -> ("NXT/EV3"=w378:T3)
          }
          frame 1 {
            (unwired) u16 1000 ("Duration (500 ms)")
            w387 = T5 2 items=["Port A"=0, "Port B"=1, "Port C"=2, "Ports A & B"=4, "Ports A & C"=5, "Ports B & C"=6, "All Ports"=3] ("Output Ports (A & B)")
            w388 = T5 4 items=["Port A"=0, "Port B"=1, "Port C"=2, "Ports A & B"=4, "Ports A & C"=5, "Ports B & C"=6, "All Ports"=3] ("Output Ports (A & B) 12")
            # "Attack Wheel"
            # "F.  Right"
            n129 = call <vilib>:"SteeringOn.vi"("Power (75)"=100, "Steering (100)"=-100, "NXT/EV3"=w381, "Output Ports (A & B)"=w387) -> ("NXT/EV3"=w384:T3)
            n130 = call <vilib>:"Wait_Num(msec).vi"("Time (100 msec)"=u32 1000, "NXT/EV3"=w384) -> ()  [unwired: 2 in, 1 out]
            n131 = call <vilib>:"SteeringOn.vi"("Power (75)"=80, "Steering (100)"=10, "NXT/EV3"=w381, "Output Ports (A & B)"=w388) -> ("NXT/EV3"=w389:T3)
          }
          frame 16 {
            # "Halt for Victory!!"
            n132 = call <vilib>:"Wait_Num(msec).vi"("Time (100 msec)"=u32 100, "NXT/EV3"=w394) -> ("NXT/EV3"=w397:T3)  [unwired: 2 in]
            n133 = xnode "Motors"() -> ("Motor"=w400:cluster{"Port":T1, "Port":T1})
            n134 = call <vilib>:"Tone.vi"("Duration (500 ms)"=u16 2000, "NXT/EV3"=w397, "Tone (440 Hz)"=u16 50) -> ("NXT/EV3"=w396:T3)  [unwired: 1 in]
            n135 = xnode "Stop Motors"("Motors"=w400, "NXT/EV3"=w396) -> ("NXT/EV3"=w398:T3)
          }
          frame 2 {
            (unwired) u16 1000 ("Duration (500 ms)")
            w413 = T5 2 items=["Port A"=0, "Port B"=1, "Port C"=2, "Ports A & B"=4, "Ports A & C"=5, "Ports B & C"=6, "All Ports"=3] ("Output Ports (A & B)")
            w414 = T5 4 items=["Port A"=0, "Port B"=1, "Port C"=2, "Ports A & B"=4, "Ports A & C"=5, "Ports B & C"=6, "All Ports"=3] ("Output Ports (A & B) 10")
            # "Attack Wheel"
            # "0 = Forward"
            n136 = call <vilib>:"SteeringOn.vi"("Power (75)"=100, "Steering (100)"=-100, "NXT/EV3"=w408, "Output Ports (A & B)"=w413) -> ("NXT/EV3"=w410:T3)
            n137 = call <vilib>:"Wait_Num(msec).vi"("Time (100 msec)"=u32 1000, "NXT/EV3"=w410) -> ()  [unwired: 2 in, 1 out]
            n138 = call <vilib>:"SteeringOn.vi"("Power (75)"=100, "Steering (100)"=0, "NXT/EV3"=w408, "Output Ports (A & B)"=w414) -> ("NXT/EV3"=w415:T3)
          }
        }
      }
    }
    n139 = Add(x=w5, y=0) -> (x+y=w3:i32)
    n140 = Not Equal To 0?(x=w3) -> (x != 0?=w2:bool)
  }
